vi "Abort handler.vi"(8 "error in (no error)":errorcluster, 10 "Logging queue element in":T2 {"Frame Size" items=["100X100"=100, "128X128"=128, "200X200"=200, "256X256"=256, "512X512"=512, "1024x1024"=1024, "2048x2048"=2048]; "Dwell time (us)" format="%#.6g"}, 11 "Logging queue in":T1) -> (0 "error out":errorcluster, 2 "Logging queue metadata shift out":T2 {"Frame Size" items=["100X100"=100, "128X128"=128, "200X200"=200, "256X256"=256, "512X512"=512, "1024x1024"=1024, "2048x2048"=2048]; "Dwell time (us)" format="%#.6g"}, 3 "Logging queue out":T1)   [LabVIEW 2013]
uses:
  Typedefs/Logging queue element.ctl
  Typedefs/Imaging Protocols enum.ctl
  Typedefs/Frame Size.ctl
  Typedefs/Acquired points count.ctl
  Typedefs/Data queue ref.ctl
  Typedefs/Read Write Enum.ctl
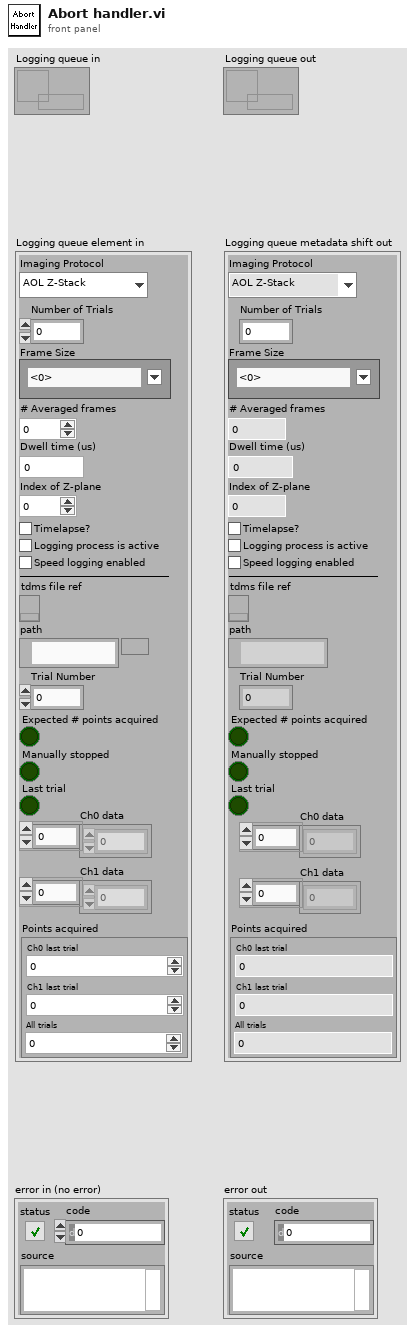
[diagram p1: front panel]
types:
  T1 = typedef "Data queue ref.ctl" = refnum<queue>
  T2 = typedef "Logging queue element.ctl" = cluster{"Imaging Protocol":T3, "Number of Trials":u16, "Frame Size":T4, "# Averaged frames":u16, "Dwell time (us)":dbl, "Index of Z-plane":i32, "Timelapse?":bool, "Logging process is active":bool, "Speed logging enabled":bool, "tdms file ref":refnum<k34>, "path":path, "Trial Number":i32, "Expected # points acquired":bool, "Manually stopped":bool, "Ch0 data":u32[], "Ch1 data":u32[], "Last trial":bool, "Points acquired":T5}
  T3 = typedef "Imaging Protocols enum.ctl" = enum16{"AOL Z-Stack", "Motor Z Stack", "Functional Acquisition", "Single Plane Acquisition", "Volume Acquisition", "Live Imaging", "Live Plane Imaging", "Live Volume Imaging"}
  T4 = typedef "Frame Size.ctl" = u16
  T5 = typedef "Acquired points count.ctl" = cluster{"Ch0 last trial":u64, "Ch1 last trial":u64, "All trials":u64}
  T6 = typedef "Read Write Enum.ctl" = enum16{"Read", "Write"}
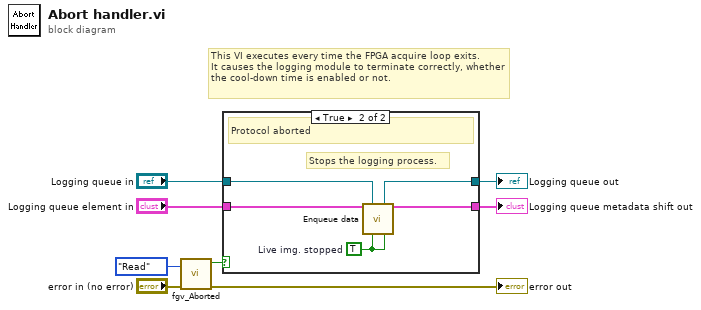
[diagram p0: block diagram]
diagram:
  # "This VI executes every time the FPGA acquire loop exits.\nIt causes the logging module to terminate correctly, whether the cool-down time is enabled or not."
  n1 = call "fgv_Aborted.vi"("error in (no error)"="error in (no error)", "Function"=Read_Write_Enum."Read") -> ("error out"=→"error out":errorcluster, "Funct Acq Aborted?"=w2:bool)  [unwired: 8 in]
  n2 = case shown="True" w2 {
    tunnel: "Logging queue in" -> [w10 w14]
    tunnel: [w10 w13] -> w4
    tunnel: [w9 w12] -> w5
    tunnel: "Logging queue element in" -> [w9 w11]
    frame False {
      # "Protocol not aborted"
    }
    frame True {
      w15 = TRUE  # Live img. stopped
      # "Stops the logging process."
      # "Protocol aborted"
      n3 = call "Enqueue data.vi"("Logging queue metadata shift in"=w11, "Logging queue in"=w14, "Expected # points acquired"=w15, "Manually stopped"=w15) -> ("Logging queue out"=w13:T1, "Logging queue metadata shift out"=w12:T2)  [unwired: 9 in, 1 out]
    }
  }
  "Logging queue metadata shift out" <- w5
  "Logging queue out" <- w4
